vi "Configure Logic Analyzer Channel.vi"(6 "Threshold Type (0: TTL)":i32(ring) items=["TTL", "CMOS", "ECL", "User"], 7 "Enable Channel State (F: Disable)":bool, 8 "error in (no error)":errorcluster, 9 "Display Position (0)":i32, 10 "Digital Channel (0: Digital 0)":i32(ring) items=["Digital 0", "Digital 1", "Digital 2", "Digital 3", "Digital 4", "Digital 5", "Digital 6", "Digital 7", "Digital 8", "Digital 9", "Digital 10", "Digital 11", "Digital 12", "Digital 13", "Digital 14", "Digital 15"], 11 "VISA resource name":refnum<visa-resource-name>) -> (0 "error out":errorcluster, 3 "VISA resource name out":refnum<visa-resource-name>)   [LabVIEW 2023, in "RIGOL DS1054Z Driver.lvlib"]
doc: "Configures the digital channel setttings for logic analyzer.\n\nNote:\nThis VI is only valid for DS1052D and DS1102D."
uses:
  <instrlib>/RIGOL-DS1054Z-LabVIEW/RIGOL DS1054Z Driver.lvlib
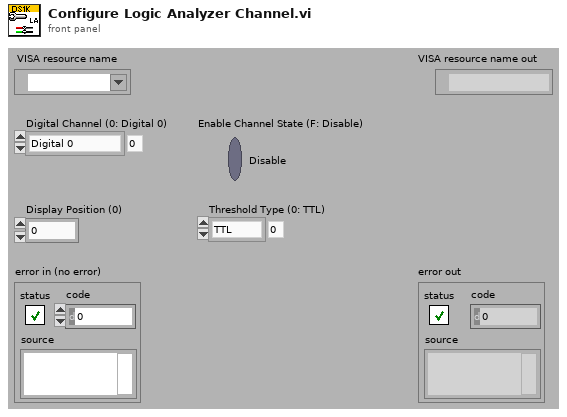
[diagram p1: front panel]
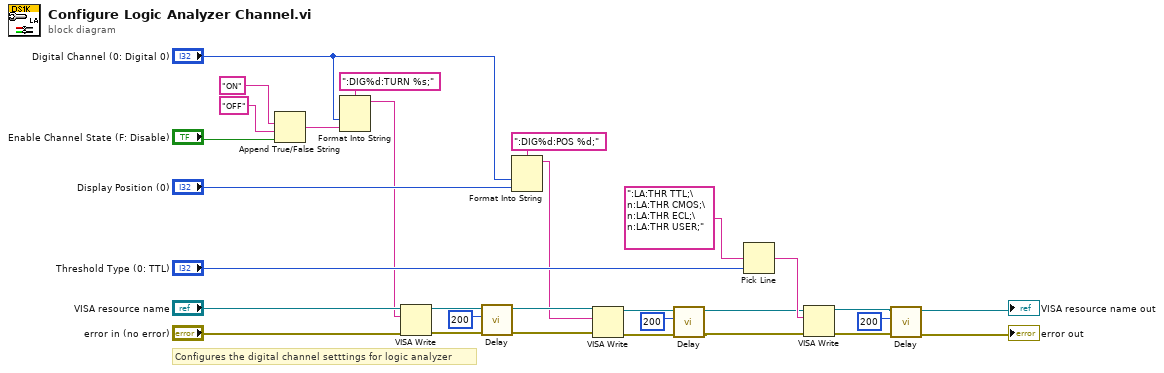
[diagram p0: block diagram]
diagram:
  # "Configures the digital channel setttings for logic analyzer"
  n1 = Append True/False String(1:"Enable Channel State (F: Disable)", 2:"OFF", 3:"ON") -> (0:w26:string)  [unwired: 1 out]
  n2 = Format Into String(format string=":DIG%d:TURN %s;", "Digital Channel (0: Digital 0)", w26) -> (resulting string=w18:string)  [unwired: 2 in, 1 out]
  n3 = VISA Write(VISA resource name="VISA resource name", write buffer=w18, error in (no error)="error in (no error)") -> (VISA resource name out=w16:refnum<visa-resource-name>, error out=w15:errorcluster)  [unwired: 1 out]
  n4 = call <instrlib>:"Delay.vi"("error in (no error)"=w15, "Delay (ms)"=u32 200, "VISA resource name"=w16) -> ("error out"=w9:errorcluster, "VISA resource name out"=w10:refnum<visa-resource-name>)  [unwired: 7 out]
  n5 = Format Into String(format string=":DIG%d:POS %d;", "Digital Channel (0: Digital 0)", "Display Position (0)") -> (resulting string=w8:string)  [unwired: 2 in, 1 out]
  n6 = VISA Write(VISA resource name=w10, write buffer=w8, error in (no error)=w9) -> (VISA resource name out=w13:refnum<visa-resource-name>, error out=w14:errorcluster)  [unwired: 1 out]
  n7 = call <instrlib>:"Delay.vi"("error in (no error)"=w14, "Delay (ms)"=u32 200, "VISA resource name"=w13) -> ("error out"=w6:errorcluster, "VISA resource name out"=w7:refnum<visa-resource-name>)  [unwired: 7 out]
  n8 = Pick Line(multi-line string=":LA:THR TTL;\n:LA:THR CMOS;\n:LA:THR ECL;\n:LA:THR USER;", line index="Threshold Type (0: TTL)") -> (output string=w21:string)  [unwired: 1 out]
  n9 = VISA Write(VISA resource name=w7, write buffer=w21, error in (no error)=w6) -> (VISA resource name out=w5:refnum<visa-resource-name>, error out=w4:errorcluster)  [unwired: 1 out]
  n10 = call <instrlib>:"Delay.vi"("error in (no error)"=w4, "Delay (ms)"=u32 200, "VISA resource name"=w5) -> ("error out"=→"error out":errorcluster, "VISA resource name out"=→"VISA resource name out":refnum<visa-resource-name>)  [unwired: 7 out]
